vi "SetSerializableData.vi"(7 "BlueSerializer in":refnum<class "BlueSerializer.lvclass">, 8 "error in (no error)":errorcluster, 10 "Data in":T1={"StructuredData"=variant(string ""), "ClassOps (child, parent)"=[]}, 11 "BlueMultiPlotConfig":refnum<class "BlueMultiPlotConfig.lvclass">) -> (0 "error out":errorcluster, 2 "Data out":T1={"StructuredData"=variant(string ""), "ClassOps (child, parent)"=[]}, 3 "BlueMultiPlotConfig":refnum<class "BlueMultiPlotConfig.lvclass">, 5 "BlueSerializer out":refnum<class "BlueSerializer.lvclass">)   [LabVIEW 2021, in "BlueMultiPlotConfig.lvclass"]
doc: "Dynamic Dispatch setter to set SerializableData for all inheritance levels of a <b>BlueSerializable</b> class. This and all overrides should ONLY be consumed by a child of <b>SerializerBase</b>"
uses:
  BlueMultiPlotConfig.lvclass
  <userlib>/Blue Origin/BlueSerialization/BlueSerializer/Support/SetSerializableDataCluster.ctl
  <userlib>/Blue Origin/BlueSerialization/BlueSerializer/Support/SetSerializableDataClusterIterable.ctl
  <userlib>/Blue Origin/BlueSerialization/BlueSerializable/BlueSerializable.lvclass
  <userlib>/Blue Origin/BlueSerialization/BlueSerializer/Support/SetSerializableDataClusterLayer.ctl
  <userlib>/Blue Origin/BlueSerialization/BlueSerializer/BlueSerializableVersion.ctl
  <userlib>/Blue Origin/BlueSerialization/BlueSerializer/Support/SetSerializableDataObject.ctl
  <userlib>/Blue Origin/BlueSerialization/BlueSerializer/BlueSerializer.lvclass
  BlueMultiPlotConfig.lvclass/BlueMultiPlotConfig.ctl
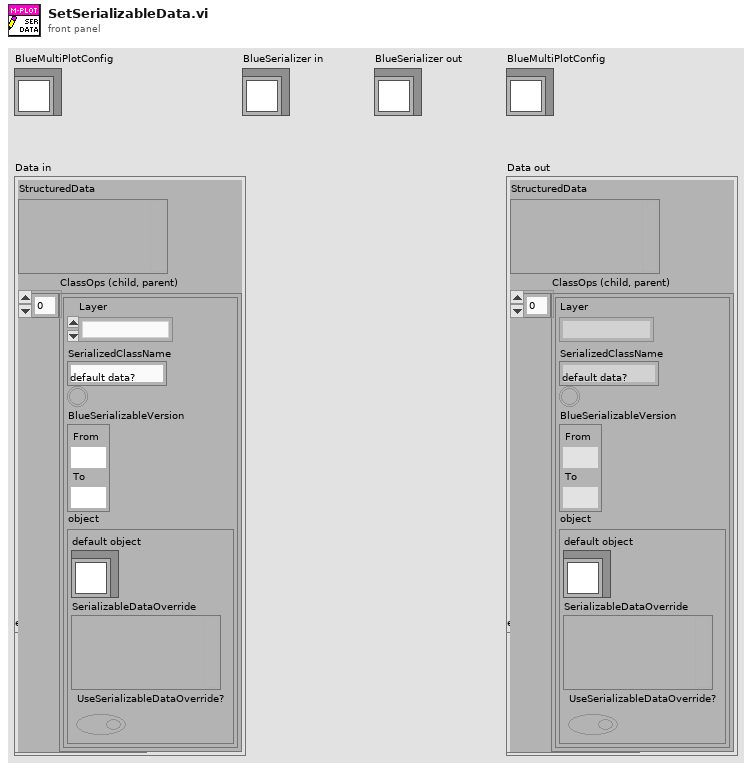
[diagram p1: front panel]
types:
  T1 = typedef "BlueSerialization.lvlib/BlueSerializer.lvclass/SetSerializableDataCluster.ctl" = cluster{"StructuredData":variant, "ClassOps (child, parent)":T2[]}
  T2 = typedef "BlueSerialization.lvlib/BlueSerializer.lvclass/SetSerializableDataClusterIterable.ctl" = cluster{"Layer":T3, "SerializedClassName":string, "default data?":bool, "BlueSerializableVersion":T4, "object":T5}
  T3 = typedef "BlueSerialization.lvlib/BlueSerializer.lvclass/SetSerializableDataClusterLayer.ctl" = enum16{"new class layer", "dropped class layer", "agreed class layer"}
  T4 = typedef "BlueSerialization.lvlib/BlueSerializer.lvclass/BlueSerializableVersion.ctl" = cluster{"From":u16, "To":u16}
  T5 = typedef "BlueSerialization.lvlib/BlueSerializer.lvclass/SetSerializableDataObject.ctl" = cluster{"default object":refnum<class "BlueSerializable.lvclass">, "SerializableDataOverride":variant, "UseSerializableDataOverride?":bool}
  T6 = typedef "BlueMultiPlotConfig.lvclass/SerializableData.ctl" = cluster{"Plots":T7[]}
  T7 = typedef "MultiStokePlot.lvlib/MultiPlotPanel.lvclass/SinglePlotConfig.ctl" = cluster{"Plot Number":i32, "Plot Bounds (%)":T8, "RocketPlotConfig":T9}
  T8 = typedef "MultiStokePlot.lvlib/MultiPlotPanel.lvclass/Window Position.ctl" = cluster{"Left (%)":dbl, "Top (%)":dbl, "Right (%)":dbl, "Bottom (%)":dbl}
  T9 = typedef "RocketPlot.lvlib/plot load data V2.ctl" = cluster{"plots":T10[], "X-axis":T12, "Y-axes":T12[], "General":T13}
  T10 = typedef "RocketPlot.lvlib/plot properties V2.ctl" = cluster{"attributes":T11, "Numeric":dbl, "Flatline?":bool}
  T11 = typedef "RocketPlot.lvlib/plot attributes V2.ctl" = cluster{"Plot Color":u32, "Point Style":u8, "Line Style":u8, "Plot Interpolation":u8, "Line Width":u8, "Bar Plot Style":u8, "Fill To":i16, "X Scale Index":u32, "Y Scale Index":u32, "Anti-aliased":bool, "Label Format":u8, "Digital Transition Type":u8, "Digital Transition Location":u8, "Digital Line Style":u8, "Fill/Point Color":u32, "Plot Name":string, "Visible":bool}
  T12 = typedef "RocketPlot.lvlib/Plot scale axis properties.ctl" = cluster{"Name Label.Text":string, "Style":u8, "Tick Colors:Minor Tick Color":u32, "Tick Colors:Tick Color":u32, "Marker Colors:Text Color":u32, "Grid Colors:Major Color":u32, "Grid Colors:Minor Color":u32, "Mapping Mode":u8, "Flipped":bool, "Name Label.Visible":bool, "Name Label.Text Colors:Text Color":u32, "Scale Fit":u8, "Range:Maximum":dbl, "Range:Minimum":dbl, "Offset and Multiplier:Multiplier":dbl, "Offset and Multiplier:Offset":dbl, "Name Label.Font:Size":u32, "Marker.Font:Size":u32, "Uniform Marker Spacing?":bool, "Format String":string}
  T13 = typedef "RocketPlot.lvlib/Plot general properties.ctl" = cluster{"Title":string, "Time to Plot":dbl, "Title.Visible":bool, "Sidebar.Visible":bool, "Plot Area:Colors:BG Color":u32, "X Scale.Plot Name":string, "X Scale.Use Plot Name":bool}
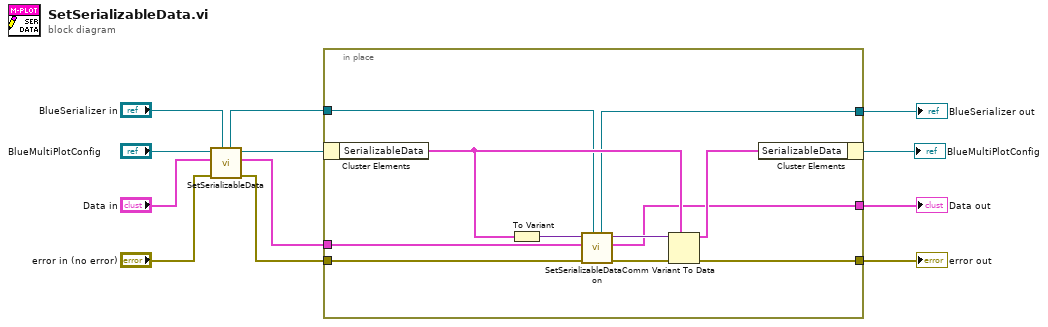
[diagram p0: block diagram]
diagram:
  n1 = call-parent "SetSerializableData.vi"("BlueSerializer in"="BlueSerializer in", "error in (no error)"="error in (no error)", "Data In"="Data in", "BlueSerializable in"="BlueMultiPlotConfig") -> ("error out"=w5:errorcluster, "Data Out"=w4:T1, "BlueSerializable out"=w3:refnum<class "BlueMultiPlotConfig.lvclass">, "BlueSerializer out"=w2:refnum<class "BlueSerializer.lvclass">)  [unwired: 4 in]
  n2 = in-place {
    in-place-border: w5 -> [w22]
    in-place-border: w2 -> [w17]
    in-place-border: [w16] -> w11
    in-place-border: [w15] -> w10
    in-place-border: [w14] -> w9
    in-place-border: w4 -> [w13]
    n3 = in-place-cluster #1(w3) -> ("SerializableData"=w19:T6)
    n4 = To Variant(anything=w19) -> (Variant=w23:variant)
    n5 = call <userlib>:"SetSerializableDataCommon.vi"("BlueSerializer in"=w17, "error in (no error)"=w22, "Data In"=w13, "SerializableData"=w23) -> ("error out"=w21:errorcluster, "Data Out"=w14:T1, "SerializableData"=w20:variant, "BlueSerializer out"=w16:refnum<class "BlueSerializer.lvclass">)  [unwired: 4 in]
    n6 = Variant To Data(error in=w21, type=w19, Variant=w20) -> (data=w18:T6, error out=w15:errorcluster)
    n7 = in-place-cluster #1("SerializableData"=w18) -> (→"BlueMultiPlotConfig":refnum<class "BlueMultiPlotConfig.lvclass">)
  }
  "error out" <- w10
  "Data out" <- w9
  "BlueSerializer out" <- w11
